vi "Inst_DS360.vi"(8 "error in":errorcluster, 10 "All Message Queues in":T1, 11 "Prueba31 in":refnum<class "Prueba32.lvclass">) -> (0 "error out":errorcluster)   [LabVIEW 2019, in "Prueba32.lvclass"]
uses:
  Prueba32.lvclass
  QMH/Message Queue/All Message Queues.ctl
  QMH/Message Queue/Message Cluster.ctl
  Prueba32.lvclass/Prueba32.ctl
  <vilib>/Utility/error.llb/Error Cluster From Error Code.vi
  QMH/Message Queue/Enqueue Message (Single).vi
  <vilib>/ErrorRing/Error Ring.xnode
  QMH/Message Queue/Message Queue.lvlib
  Instrumento/DS360/DS360.lvclass
panel:
  out "Frec (Hz)":dbl
  out "Amplitud (Vrms)":dbl
  out "All States":string[](array[string])
  out "Actual State":string
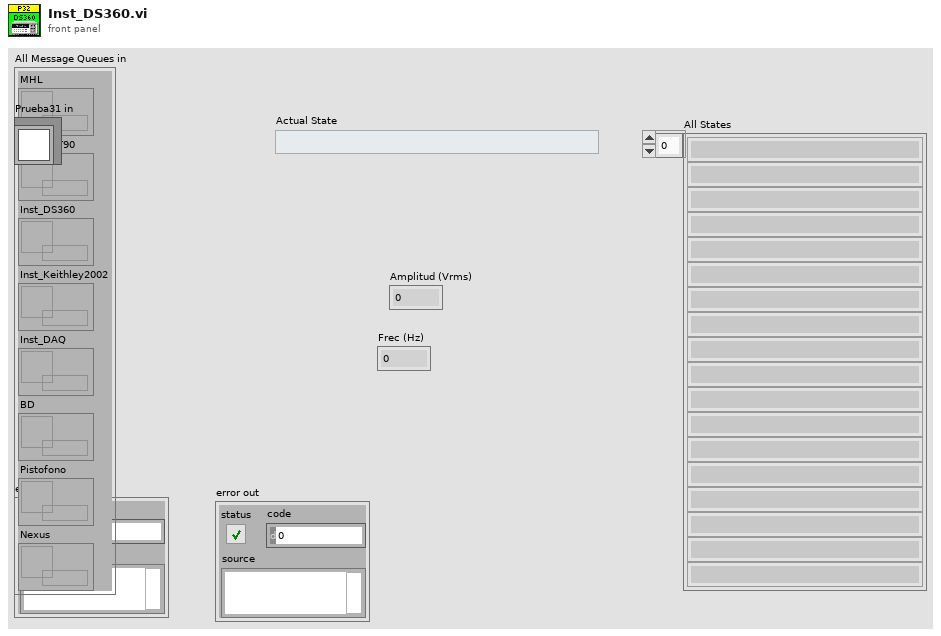
[diagram p1: front panel]
types:
  T1 = typedef "Message Queue.lvlib/All Message Queues.ctl" = cluster{"MHL":refnum<queue>, "Inst_CNT90":refnum<queue>, "Inst_DS360":refnum<queue>, "Inst_Keithley2002":refnum<queue>, "Inst_DAQ":refnum<queue>, "BD":refnum<queue>, "Pistofono":refnum<queue>, "Nexus":refnum<queue>}
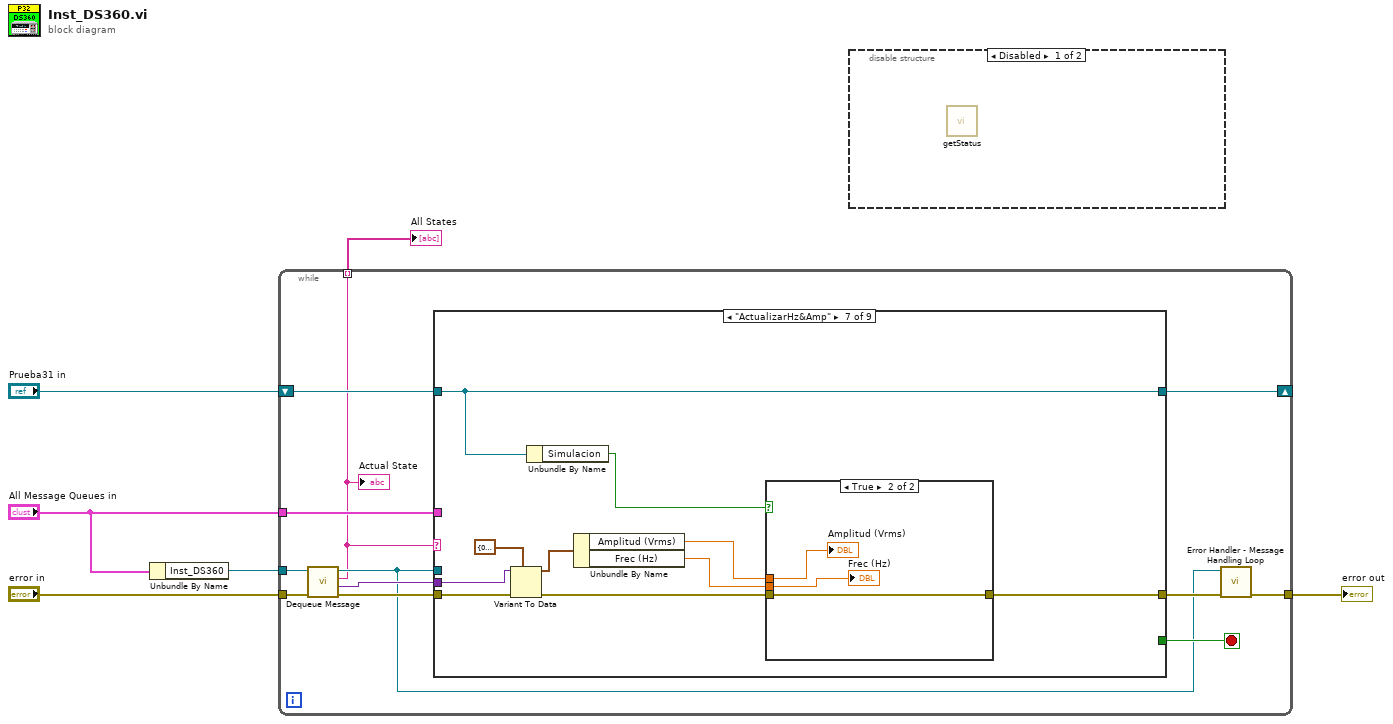
[diagram p0: block diagram]
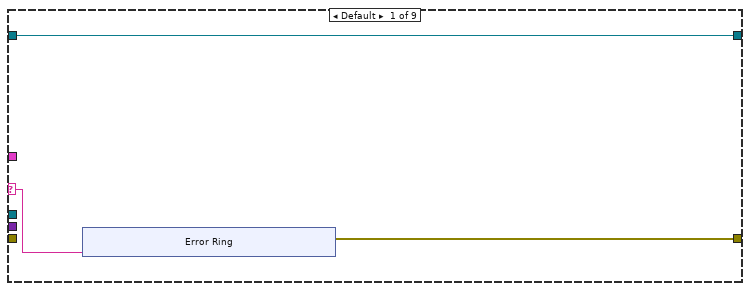
[diagram p3: hidden frame]
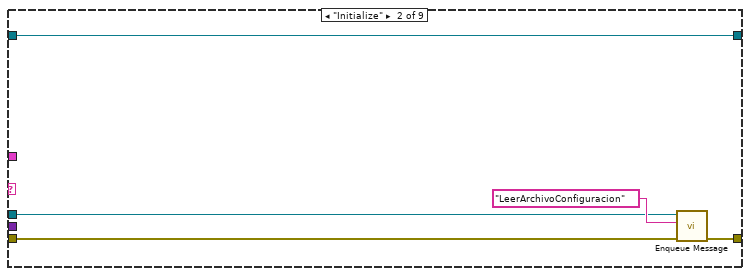
[diagram p4: hidden frame]
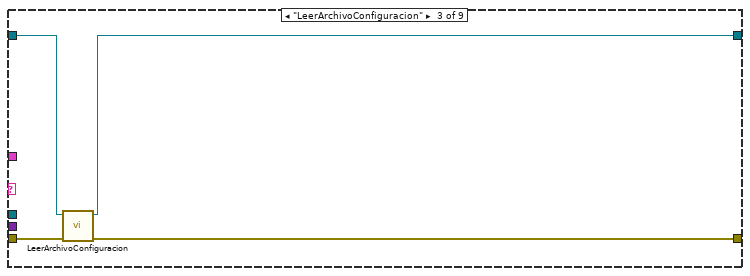
[diagram p5: hidden frame]
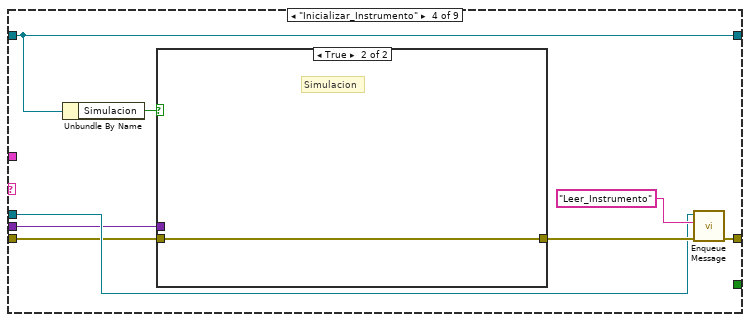
[diagram p6: hidden frame]
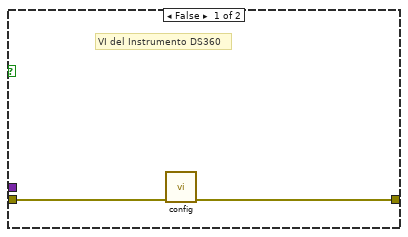
[diagram p7: hidden frame]
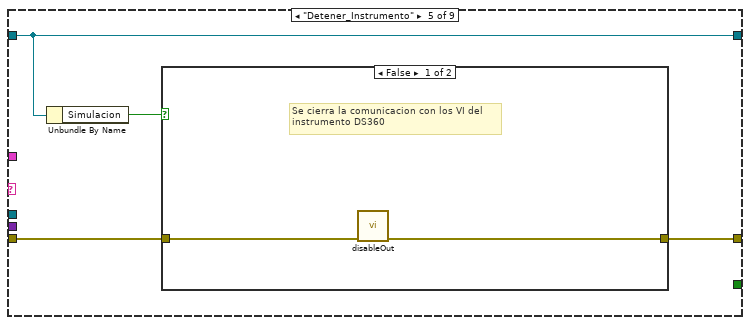
[diagram p8: hidden frame]
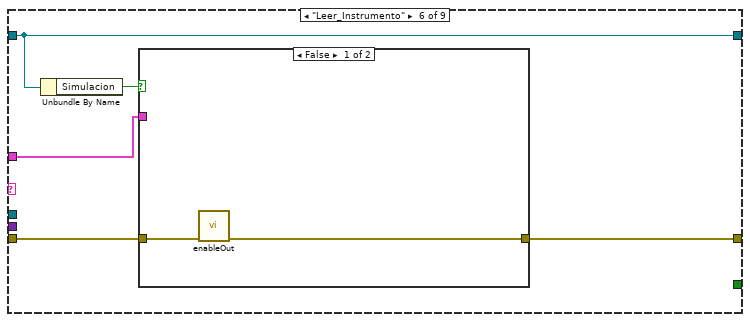
[diagram p10: hidden frame]
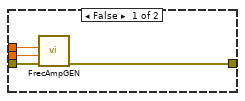
[diagram p12: hidden frame]
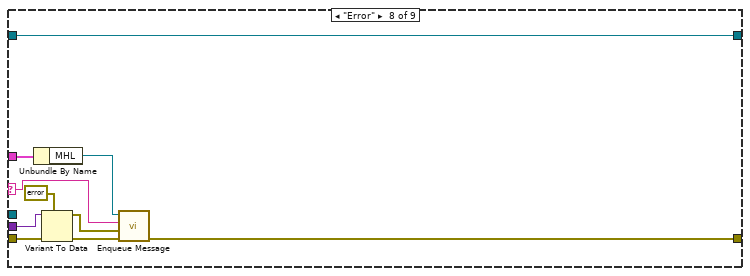
[diagram p13: hidden frame]
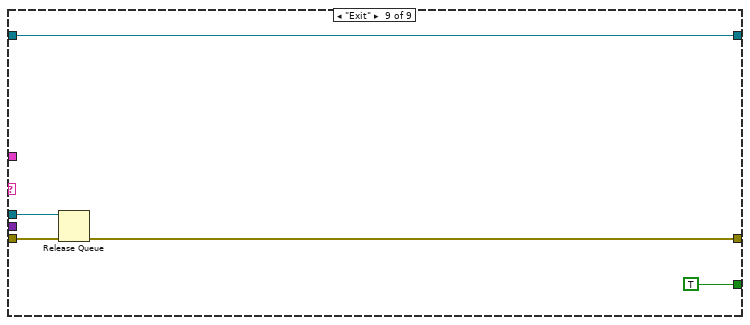
[diagram p14: hidden frame]
diagram:
  n1 = Unbundle By Name("All Message Queues in") -> ("Inst_DS360"=w4:refnum<queue>)
  n2 = while {
    tunnel: "error in" -> [w18]
    tunnel: w4 -> [w17]
    tunnel: "All Message Queues in" -> [w16]
    tunnel: [w9] -> w2
    shift-right: [w12] -> _
    shift-left: "Prueba31 in" -> [w15]
    tunnel: [w7] -> w1 mode=indexing
    stop <- w11 stop-if-true
    n3 = call "Dequeue Message.vi"("error in (no error)"=w18, "Message Queue"=w17) -> ("error out"=w13:errorcluster, "Message Data"=w14:variant, "Message"=w7:string, "dup Message Queue"=w8:refnum<queue>)  [unwired: 6 in]
    "Actual State" <- w7
    n4 = case shown="\"ActualizarHz&Amp\"" w7 {
      selector: w7 -> [w21 _ _ _ _ _ _ w83 _]
      tunnel: w16 -> [_ _ _ _ _ w59 _ w82 _]
      tunnel: w15 -> [w19 w33 w34 w42 w51 w58 w65 w90 w92]
      tunnel: w8 -> [_ w29 _ w41 _ _ _ _ w94]
      tunnel: w14 -> [_ _ _ w40 _ _ w70 w87 _]
      tunnel: w13 -> [_ w30 w36 w39 w49 w60 w71 w88 w95]
      tunnel: [w20 w31 w37 w38 w52 w56 w73 w85 w91] -> w10
      tunnel: [w19 w33 w35 w42 w51 w58 w65 w90 w92] -> w12
      tunnel: [_ _ _ _ _ _ _ _ TRUE] -> w11
      frame Default {
        n5 = xnode "Error Ring"("parameter 0"=w21) -> ("error out"=w20:errorcluster)
      }
      frame "Initialize" {
        n6 = call-poly "Enqueue Message.vi"("error in (no error)"=w30, "Message"="LeerArchivoConfiguracion", "Message Queue"=w29) -> ("error out"=w31:errorcluster)  [unwired: 7 in, 1 out]
      }
      frame "LeerArchivoConfiguracion" {
        n7 = call "LeerArchivoConfiguracion.vi"("error in"=w36, "Prueba31 in"=w34) -> ("error out"=w37:errorcluster, "Prueba31 out"=w35:refnum<class "Prueba32.lvclass">)  [unwired: 8 in]
      }
      frame "Inicializar_Instrumento" {
        n8 = Unbundle By Name(w42) -> ("Simulacion"=w44:bool)
        n9 = case shown="True" w44 {
          tunnel: [w47 w48] -> w45
          tunnel: w39 -> [w46 w48]
          tunnel: w40 -> [_ _]
          frame False {
            # "VI del Instrumento DS360"
            n10 = call "config.vi"("error in (no error)"=w46) -> ("error out"=w47:errorcluster)  [unwired: 9 in, 1 out]
          }
          frame True {
            # "Simulacion"
          }
        }
        n11 = call-poly "Enqueue Message.vi"("error in (no error)"=w45, "Message"="Leer_Instrumento", "Message Queue"=w41) -> ("error out"=w38:errorcluster)  [unwired: 7 in, 1 out]
      }
      frame "Detener_Instrumento" {
        n12 = Unbundle By Name(w51) -> ("Simulacion"=w50:bool)
        n13 = case shown="False" w50 {
          tunnel: [w54 w55] -> w52
          tunnel: w49 -> [w53 w55]
          frame False {
            # "Se cierra la comunicacion con los VI del\ninstrumento DS360"
            n14 = call "disableOut.vi"("error in (no error)"=w53) -> ("error out"=w54:errorcluster)  [unwired: 9 in, 1 out]
          }
          frame True {
            # "Simulacion"
          }
        }
      }
      frame "Leer_Instrumento" {
        n15 = Unbundle By Name(w58) -> ("Simulacion"=w57:bool)
        n16 = case shown="False" w57 {
          tunnel: [w61 w63] -> w56
          tunnel: w60 -> [w62 w63]
          tunnel: w59 -> [_ _]
          frame False {
            n17 = call "enableOut.vi"("error in (no error)"=w62) -> ("error out"=w61:errorcluster)  [unwired: 9 in, 1 out]
          }
          frame True {
          }
        }
      }
      frame "ActualizarHz&Amp" {
        n18 = Variant To Data(error in=w71, type=cluster{"Amplitud (Vrms)":dbl, "Frec (Hz)":dbl} {"Amplitud (Vrms)"=0.0, "Frec (Hz)"=0.0}, Variant=w70) -> (data=w68:cluster{"Amplitud (Vrms)":dbl, "Frec (Hz)":dbl}, error out=w72:errorcluster)
        n19 = Unbundle By Name(w65) -> ("Simulacion"=w64:bool)
        n20 = Unbundle By Name(w68) -> ("Amplitud (Vrms)"=w66:dbl, "Frec (Hz)"=w67:dbl)
        n21 = case shown="True" w64 {
          tunnel: [w77 w80] -> w73
          tunnel: w72 -> [w76 w80]
          tunnel: w67 -> [w75 w78]
          tunnel: w66 -> [w74 w79]
          frame False {
            n22 = call "FrecAmpGEN.vi"("error in (no error)"=w76, "Frec (Hz)"=w75, "Amplitud (Vrms)"=w74) -> ("error out"=w77:errorcluster)  [unwired: 7 in, 1 out]
          }
          frame True {
            "Amplitud (Vrms)" <- w79
            "Frec (Hz)" <- w78
          }
        }
      }
      frame "Error" {
        n23 = Unbundle By Name(w82) -> ("MHL"=w81:refnum<queue>)
        n24 = Variant To Data(error in=w88, type=errorcluster {"status"=FALSE, "code"=0, "source"=""} ("error constant"), Variant=w87) -> (data=w84:errorcluster, error out=w86:errorcluster)
        n25 = call-poly "Enqueue Message.vi"("error in (no error)"=w86, "Message Data"=w84, "Message"=w83, "Message Queue"=w81) -> ("error out"=w85:errorcluster)  [unwired: 6 in, 1 out]
      }
      frame "Exit" {
        n26 = Release Queue(queue=w94, error in (no error)=w95) -> (error out=w91:errorcluster)  [unwired: 1 in, 2 out]
      }
    }
    n27 = call "Error Handler - Message Handling Loop.vi"("error in (no error)"=w10, "Message Queue"=w8) -> ("dup error in"=w9:errorcluster)  [unwired: 8 in, 1 out]
  }
  "error out" <- w2
  "All States" <- w1
  n28 = disable-structure shown="Disabled" {
    frame Disabled {
      n29 = call "getStatus.vi"() -> ()  [unwired: 9 in, 3 out]
    }
    frame Enabled {
    }
  }
